vi "Sort Array (I16).vi"(6 "Max Size":i32=200, 10 "New Element":i16, 11 "Array In":i16[](array[numeric])) -> (3 "Array Out":i16[](array[numeric]))   [LabVIEW 2015]
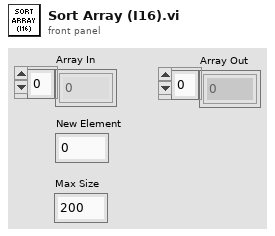
[diagram p1: front panel]
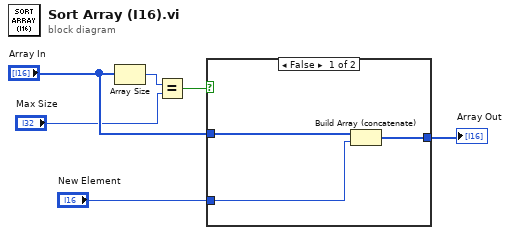
[diagram p0: block diagram]
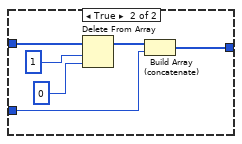
[diagram p2: hidden frame]
diagram:
  n1 = Array Size(array="Array In") -> (size(s)=w5:i32)
  n2 = Equal?(x=w5, y="Max Size") -> (x = y?=w3:bool)
  n3 = case shown="False" w3 {
    tunnel: "Array In" -> [w9 w15]
    tunnel: [w8 w11] -> w1
    tunnel: "New Element" -> [w7 w10]
    frame False {
      n4 = Build Array (concatenate)(w9, w7) -> (w8:i16[])
    }
    frame True {
      n5 = Delete From Array(array=w15, length=1, index=0) -> (array with subset deleted=w12:i16[])  [unwired: 1 out]
      n6 = Build Array (concatenate)(w12, w10) -> (w11:i16[])
    }
  }
  "Array Out" <- w1
